vi "svm_remove_model_padding.vi"(8 "error in (no error)":errorcluster, 11 "Padded model":T6) -> (0 "error out":errorcluster, 3 "Model":T1)   [LabVIEW 2015]
uses:
  Controls/svm_model_padded.ctl
  Controls/svm_parameter.ctl
  Controls/svm_type.ctl
  Controls/svm_kernel_type.ctl
  Controls/svm_node_padded.ctl
  Controls/svm_model.ctl
  Controls/svm_node.ctl
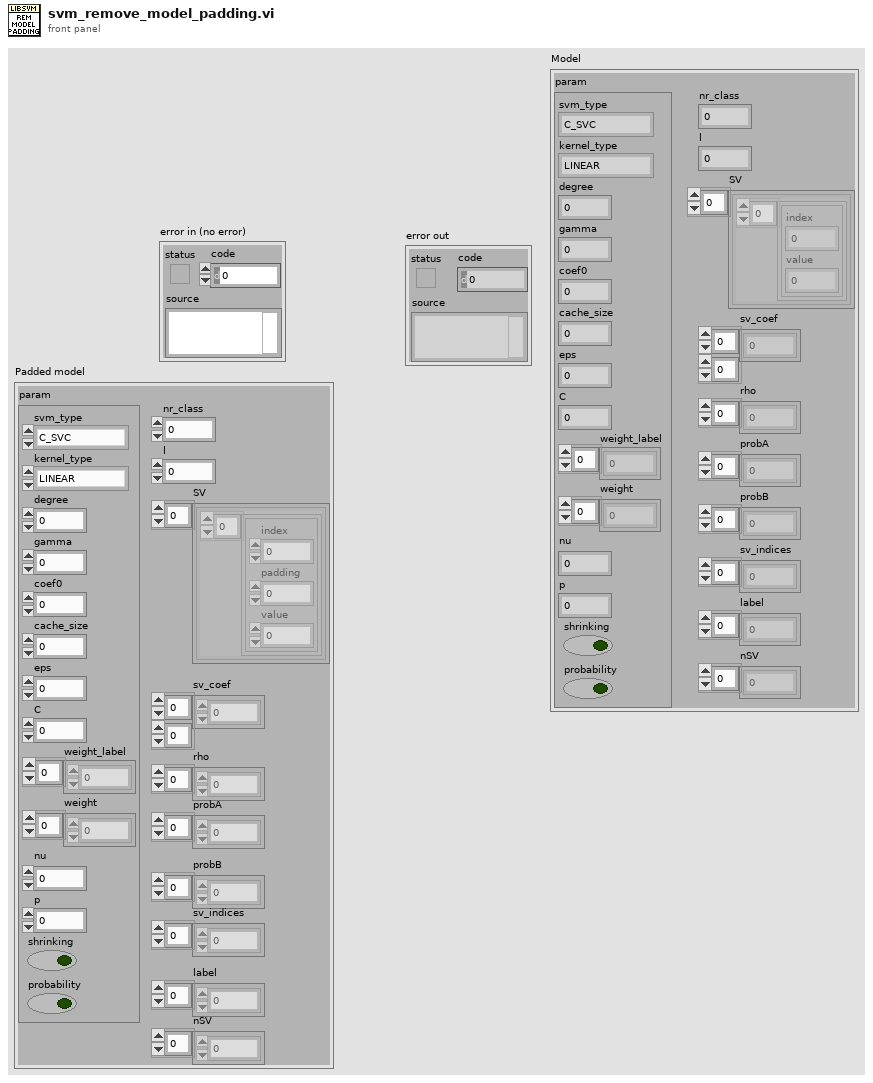
[diagram p1: front panel]
types:
  T1 = typedef "svm_model.ctl" = cluster{"param":T2, "nr_class":i32, "l":i32, "SV":cluster{"Array":T5[]}[], "sv_coef":dbl[][], "rho":dbl[], "probA":dbl[], "probB":dbl[], "sv_indices":i32[], "label":i32[], "nSV":i32[]}
  T2 = typedef "svm_parameter.ctl" = cluster{"svm_type":T3, "kernel_type":T4, "degree":i32, "gamma":dbl, "coef0":dbl, "cache_size":dbl, "eps":dbl, "C":dbl, "weight_label":i32[], "weight":dbl[], "nu":dbl, "p":dbl, "shrinking":bool, "probability":bool}
  T3 = typedef "svm_type.ctl" = enum32{"C_SVC", "NU_SVC", "ONE_CLASS", "EPSILON_SVR", "NU_SVR"}
  T4 = typedef "svm_kernel_type.ctl" = enum32{"LINEAR", "POLY", "RBF", "SIGMOID", "PRECOMPUTED"}
  T5 = typedef "svm_node.ctl" = cluster{"index":i32, "value":dbl}
  T6 = typedef "svm_model_padded.ctl" = cluster{"param":T2, "nr_class":i32, "l":i32, "SV":cluster{"Array":T7[]}[], "sv_coef":dbl[][], "rho":dbl[], "probA":dbl[], "probB":dbl[], "sv_indices":i32[], "label":i32[], "nSV":i32[]}
  T7 = typedef "svm_node_padded.ctl" = cluster{"index":i32, "padding":i32, "value":dbl}
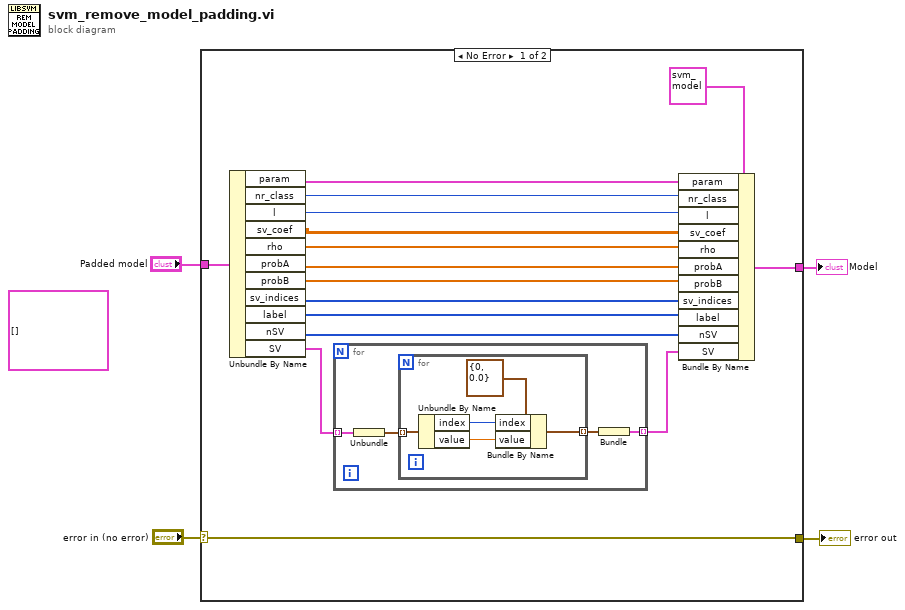
[diagram p0: block diagram]
diagram:
  (unwired) cluster{"Array":T7[]}[] [] ("SV")
  n1 = case shown="No Error" "error in (no error)" {
    selector: "error in (no error)" -> [w7 w30]
    tunnel: [w7 w30] -> w4
    tunnel: "Padded model" -> [w20 _]
    tunnel: [w18 _] -> w1
    frame No Error {
      n2 = Unbundle By Name(w20) -> ("param"=w17:T2, "nr_class"=w16:i32, "l"=w15:i32, "sv_coef"=w14:dbl[][], "rho"=w13:dbl[], "probA"=w12:dbl[], "probB"=w11:dbl[], "sv_indices"=w10:i32[], "label"=w9:i32[], "nSV"=w8:i32[], "SV"=w6:cluster{"Array":T7[]}[])
      n3 = for {
        tunnel: w6 -> [w24] mode=indexing
        tunnel: [w21] -> w5 mode=indexing
        n4 = Unbundle(w24) -> ("Array"=w23:T7[])
        n5 = for {
          tunnel: w23 -> [w29] mode=indexing
          tunnel: [w25] -> w22 mode=indexing
          n6 = Unbundle By Name(w29) -> ("index"=w27:i32, "value"=w26:dbl)
          n7 = Bundle By Name(cluster=T5 {"index"=0, "value"=0.0} ("svm_node"), "index"=w27, "value"=w26) -> (w25:T5)
        }
        n8 = Bundle(w22) -> (w21:cluster{T5[]})  [unwired: 1 in]
      }
      n9 = Bundle By Name(cluster=T1 {"param"={"svm_type"=enum."C_SVC", "kernel_type"=enum."LINEAR", "degree"=0, "gamma"=0.0, "coef0"=0.0, "cache_size"=0.0, "eps"=0.0, "C"=0.0, "weight_label"=[], "weight"=[], "nu"=0.0, "p"=0.0, "shrinking"=FALSE, "probability"=FALSE}, "nr_class"=0, "l"=0, "SV"=[], "sv_coef"=[], "rho"=[], "probA"=[], "probB"=[], "sv_indices"=[], "label"=[], "nSV"=[]} ("svm_model"), "param"=w17, "nr_class"=w16, "l"=w15, "sv_coef"=w14, "rho"=w13, "probA"=w12, "probB"=w11, "sv_indices"=w10, "label"=w9, "nSV"=w8, "SV"=w5) -> (w18:T1)
    }
    frame Error {
    }
  }
  "error out" <- w4
  "Model" <- w1
